vi "FindAck.vi"(7 "ack":refnum<k4>, 10 "parms in":T2={"subchannel"=0, "size (0)"=0, "abort (F)"=FALSE, "timeout"=-1, "ack id (0)"=0, "last elt? (F)"=FALSE, "valid? (T)"=FALSE, "GUID"=""}, 11 "MessengerMCPU in":refnum<class "MessengerMCPU.lvclass">) -> (1 "wait":bool, 2 "parms out":T1, 3 "MessengerMCPU out":refnum<class "MessengerMCPU.lvclass">)   [LabVIEW 2019, in "MessengerM.lvlib" / "MessengerMCPU.lvclass"]
uses:
  MessengerMCPU.lvclass
  ParmsOut.ctl
  MessengerM.lvlib
  ParmsIn.ctl
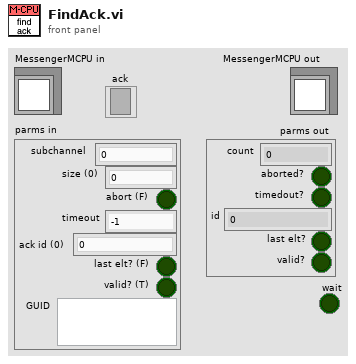
[diagram p1: front panel]
types:
  T1 = typedef "MessengerM.lvlib/ParmsOut.ctl" = cluster{"count":i32, "aborted?":bool, "timedout?":bool, "id":u32, "last elt?":bool, "valid?":bool}
  T2 = typedef "MessengerM.lvlib/ParmsIn.ctl" = cluster{"subchannel":i32, "size (0)":i32, "abort (F)":bool, "timeout":i32, "ack id (0)":u32, "last elt? (F)":bool, "valid? (T)":bool, "GUID":string}
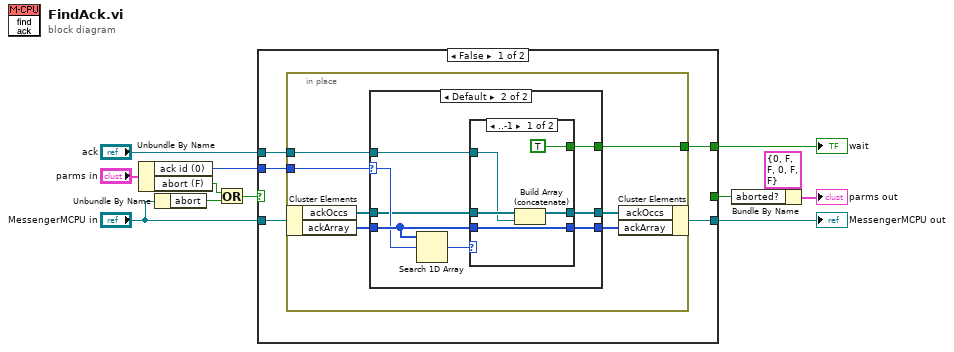
[diagram p0: block diagram]
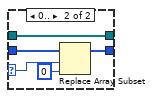
[diagram p3: hidden frame]
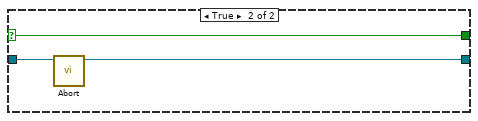
[diagram p4: hidden frame]
diagram:
  n1 = Unbundle By Name("parms in") -> ("ack id (0)"=w4:u32, "abort (F)"=w5:bool)
  n2 = Unbundle By Name("MessengerMCPU in") -> ("abort"=w9:bool)
  n3 = Or(x=w5, y=w9) -> (x .or. y?=w8:bool)
  n4 = case shown="False" w8 {
    selector: w8 -> [_ w45]
    tunnel: "MessengerMCPU in" -> [w17 w47]
    tunnel: [w16 w46] -> w12
    tunnel: [w15 _] -> w11
    tunnel: [_ w45] -> w2
    tunnel: "ack" -> [w14 _]
    tunnel: w4 -> [w13 _]
    frame False {
      n5 = in-place {
        in-place-border: [w22] -> w15
        in-place-border: w14 -> [w19]
        in-place-border: w13 -> [w18]
        n6 = in-place-cluster #1(w17) -> ("ackOccs"=w20:refnum<k4>[], "ackArray"=w24:u32[])
        n7 = case shown="Default" w18 {
          selector: w18 -> [_ w30]
          tunnel: [_ w34] -> w22
          tunnel: w24 -> [w26 w33]
          tunnel: [w26 w32] -> w23
          tunnel: [w25 w29] -> w21
          tunnel: w20 -> [w25 w28]
          tunnel: w19 -> [_ w27]
          frame 0 {
          }
          frame Default {
            n8 = Search 1D Array(1D array=w33, element=w30) -> (index of element=w31:i32)  [unwired: 1 in]
            n9 = case shown="..-1" w31 {
              selector: w31 -> [_ w42]
              tunnel: [w39 w43] -> w32
              tunnel: w33 -> [w39 w44]
              tunnel: [TRUE _] -> w34
              tunnel: [w36 w40] -> w29
              tunnel: w28 -> [w37 w40]
              tunnel: w27 -> [w35 _]
              frame ..-1 {
                n10 = Build Array (concatenate)(w37, w35) -> (w36:refnum<k4>[])
              }
              frame 0.. {
                n11 = Replace Array Subset(array=w44, new element=u32 0 ("new element/subarray"), index=w42) -> (w43:u32[])
              }
            }
          }
        }
        n12 = in-place-cluster #1("ackOccs"=w21, "ackArray"=w23) -> (w16:refnum<class "MessengerMCPU.lvclass">)
      }
    }
    frame True {
      n13 = call-dynamic "Abort.vi"("MessengerMCPU in"=w47) -> ("MessengerMCPU out"=w46:refnum<class "MessengerMCPU.lvclass">)  [unwired: 10 in]
    }
  }
  "MessengerMCPU out" <- w12
  "wait" <- w11
  n14 = Bundle By Name(cluster=T1 {"count"=0, "aborted?"=FALSE, "timedout?"=FALSE, "id"=0, "last elt?"=FALSE, "valid?"=FALSE} ("parms out"), "aborted?"=w2) -> (→"parms out":T1)
